vi "get Recent User List.vi"(5 "[Data] Recent User in":refnum<class "[User] Recent Login.lvclass">) -> (2 "recent user list":string[](array[string]))   [LabVIEW 2020, in "[User] Recent Login.lvclass"]
uses:
  [User] Recent Login.lvclass
  [User] Recent Login.lvclass/[User] Recent Login.ctl
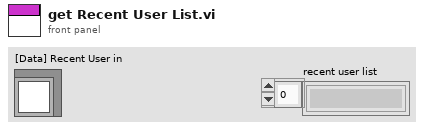
[diagram p1: front panel]
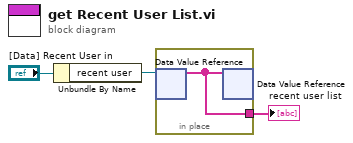
[diagram p0: block diagram]
diagram:
  n1 = Unbundle By Name("[Data] Recent User in") -> ("recent user"=w1:refnum<data-value>)
  n2 = in-place {
    in-place-border: [w4] -> w2
    n3 = in-place-dvr #1(w1) -> (w4:string[])  [unwired: 1 out]
    n4 = in-place-dvr #1(w4) -> ()  [unwired: 2 out]
  }
  "recent user list" <- w2
